vi "Dateischreiben_Echtes_Signal_ohneExcel.vi"() -> ()   [LabVIEW 2016]
panel:
  out "PT":dbl
  out "Te":dbl
  in  "Messfrequenz":dbl=10.0
  out "Signalverlaufsdiagramm 2":dynamicdata(graph)
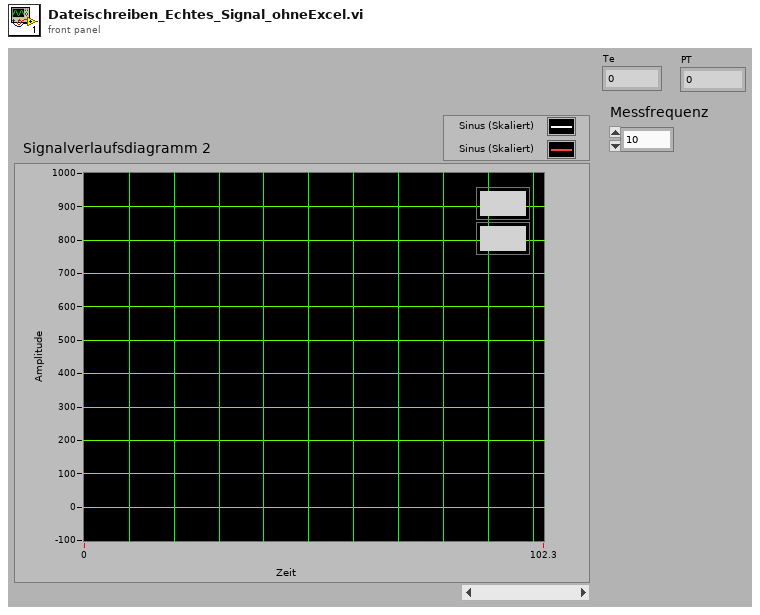
[diagram p1: front panel]
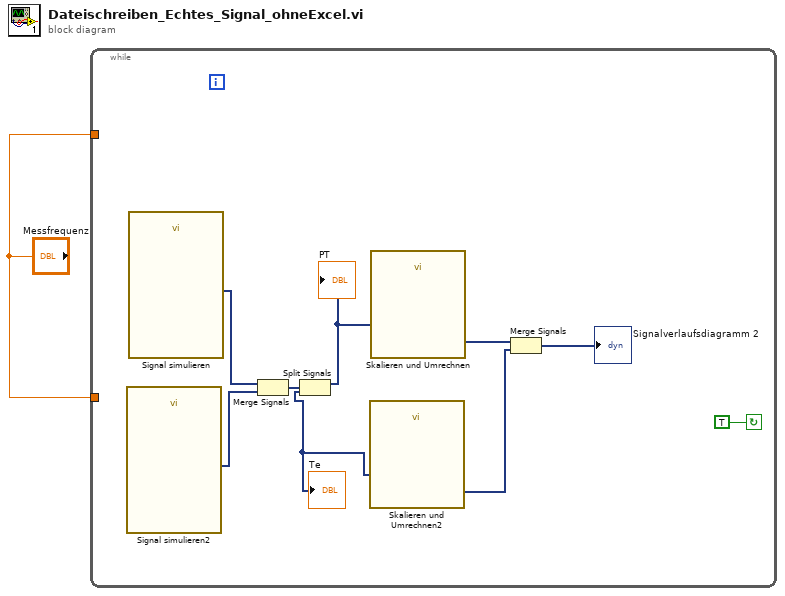
[diagram p0: block diagram]
diagram:
  n1 = while {
    tunnel: "Messfrequenz" -> [_]
    tunnel: "Messfrequenz" -> [_]
    stop <- TRUE continue-if-true
    n2 = call "Signal simulieren2"() -> ("Sinus"=w7:dynamicdata)  [unwired: 14 in, 1 out]
    n3 = call "Signal simulieren"() -> ("Sinus"=w8:dynamicdata)  [unwired: 14 in, 1 out]
    n4 = Merge Signals(w8, w7) -> (w6:dynamicdata)
    n5 = Split Signals(w6) -> (w3:dynamicdata, w2:dynamicdata)  [unwired: 2 in]
    "Te" <- w2
    "PT" <- w3
    n6 = call "Skalieren und Umrechnen2"("Signals"=w2) -> ("Scaled Signals"=w4:dynamicdata)  [unwired: 9 in, 1 out]
    n7 = call "Skalieren und Umrechnen"("Signals"=w3) -> ("Scaled Signals"=w9:dynamicdata)  [unwired: 9 in, 1 out]
    n8 = Merge Signals(w9, w4) -> (→"Signalverlaufsdiagramm 2":dynamicdata)
  }
